vi "number1-cannonball.vi"() -> ()   [LabVIEW 2014]
panel:
  in  "threshold of energy remained for the cannonball not bouncing again (%)":dbl
  in  "energy loss (%)":dbl
  in  "initial angle":dbl
  in  "initial velocity":dbl
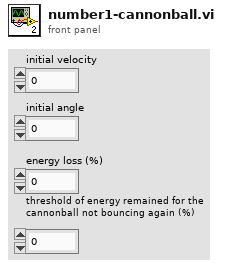
[diagram p1: front panel]
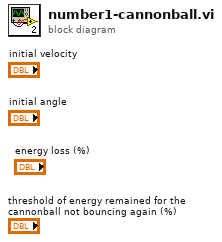
[diagram p0: block diagram]
diagram:
